vi "PcTestCode.vi"() -> ()   [LabVIEW 2020]
panel:
  in  "error in":errorcluster
  out "error out":errorcluster
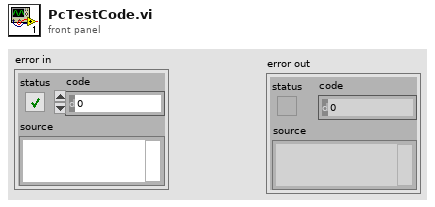
[diagram p1: front panel]
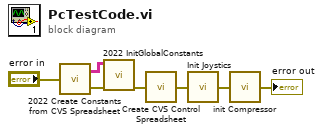
[diagram p0: block diagram]
diagram:
  n1 = call "2022 Create Constants from CVS Spreadsheet.vi"("error in"="error in") -> ("localConstantSpreadSheet"=w6:string[][], "error out"=w5:errorcluster)
  n2 = call "2022 InitGlobalConstants.vi"("error in (no error)"=w5, "localConstantSpreadSheet"=w6) -> ("error out"=w2:errorcluster)  [unwired: 9 in]
  n3 = call "Create CVS Control Spreadsheet.vi"("error in"=w2) -> ("error out"=w1:errorcluster)
  n4 = call "Init Joystics.vi"("error in"=w1) -> ("error out"=w4:errorcluster)
  n5 = call "init Compressor.vi"("error in (no error)"=w4) -> ("error out"=→"error out":errorcluster)
